vi "Payload to Word.vi"(3 "Payload":string) -> (1 "Word":i16[](array[numeric]))   [LabVIEW 2019]
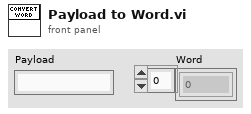
[diagram p1: front panel]
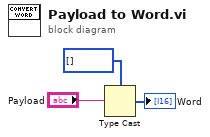
[diagram p0: block diagram]
diagram:
  n1 = Type Cast(type=i16[] [] ("Data"), x="Payload") -> (*(type *) &x=→"Word":i16[])
